vi "InitClass.vi"(11 "TSM Context":T1) -> (0 "error out":errorcluster)   [LabVIEW 2019, in "GlobalTestData.lvclass"]
doc: "This function should be called once at the start of a test program (ProcessSetup). It will initialize the class data."
uses:
  GlobalTestData.lvclass
  <vilib>/NI_TestStand_SemiconductorModule/NI_TestStand_Semiconductor_Module.lvlibp/PinMap/General/SemiconductorModuleContext.ctl
  GlobalTestData.lvclass/GlobalTestData.ctl
  Private/PersistantClassData.vi
  <vilib>/NI_TestStand_SemiconductorModule/NI_TestStand_Semiconductor_Module.lvlibp
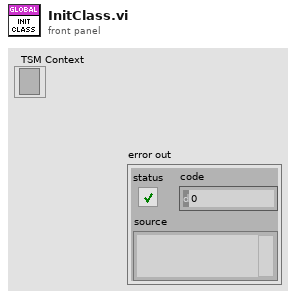
[diagram p1: front panel]
types:
  T1 = typedef "NI_TestStand_Semiconductor_Module.lvlibp/SemiconductorModuleContext.ctl" = refnum<k7>
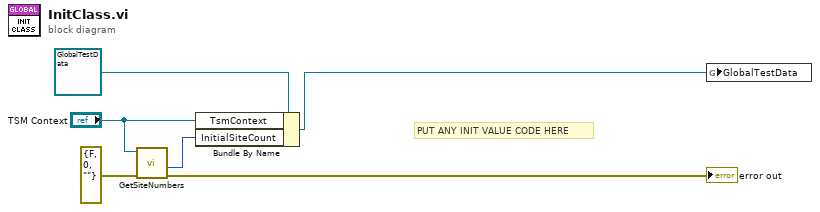
[diagram p0: block diagram]
diagram:
  # "PUT ANY INIT VALUE CODE HERE"
  n1 = call <vilib>:"GetSiteNumbers.vi"("error in (no error)"=errorcluster {"status"=FALSE, "code"=0, "source"=""} ("error out"), "Semiconductor Module Context"="TSM Context") -> ("error out"=→"error out":errorcluster, "Number Of Sites"=w1:i32)  [unwired: 6 in, 2 out]
  n2 = Bundle By Name(cluster=refnum<class "GlobalTestData.lvclass"> refnum ("GlobalTestData"), "TsmContext"="TSM Context", "InitialSiteCount"=w1) -> (w4:refnum<class "GlobalTestData.lvclass">)
  n3 = global write "PersistantClassData.vi" "GlobalTestData"(w4) -> ()
